vi "FourSessThreePinTwoInstrTwoSiteReservation_CallGetConnectionsFromPinsForOneFgenPinAllSites_ReturnsOneConnection.vi"(8 "error in":errorcluster) -> (0 "error out":errorcluster, 2 "result":string, 3 "pass":bool)   [LabVIEW 2020, in "MeasurementServerTests.lvlib"]
uses:
  MeasurementServerTests.lvlib
  Runtime/MeasurementLink Session Management/Session Reservation/Connection.ctl
  Runtime/MeasurementLink Session Management/Session Reservation/Hardware Independent Connection.ctl
  c3cb69a0-23cd-49fc-99d1-8c54773f0200.vi
  b3e5c3be-b7a7-4b6e-86ee-709eea9cb752.vi
  Runtime/MeasurementLink Session Management/Session Reservation/Get Connections Impl.vi
  Runtime/MeasurementLink Session Management/Session Reservation/Session Reservation.lvclass
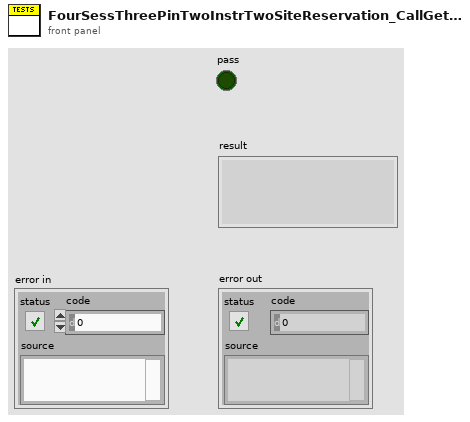
[diagram p1: front panel]
types:
  T1 = typedef "MeasurementLink Session Management.lvlib/Session Reservation.lvclass/Hardware Independent Connection.ctl" = cluster{"pin or relay name":string, "site":i32, "instrument type id":string, "channel":string}
  T2 = typedef "MeasurementLink Session Management.lvlib/Session Reservation.lvclass/Connection.ctl" = cluster{"connection":T1, "session":variant}
  T3 = typedef "MeasurementLink Session Management.lvlib/Session Reservation.lvclass/Data.ctl" = cluster{"session and driver infos":T4[], "pins":string[]}
  T4 = typedef "MeasurementLink Session Management.lvlib/Session Reservation.lvclass/Session and Driver Info.ctl" = cluster{"session info":T5, "session created":bool, "session":variant}
  T5 = typedef "MeasurementLink Session Management Client.lvlib/ni_measurementlink_sessionmanagement_v1_SessionInformation.ctl" = cluster{"session":T6, "resource_name":string, "channel_list":string, "instrument_type_id":string, "session_exists":bool, "channel_mappings":T7[]}
  T6 = typedef "MeasurementLink Session Management Client.lvlib/nidevice_grpc_Session.ctl" = cluster{"name":string}
  T7 = typedef "MeasurementLink Session Management Client.lvlib/ni_measurementlink_sessionmanagement_v1_ChannelMapping.ctl" = cluster{"pin_or_relay_name":string, "site":i32, "channel":string}
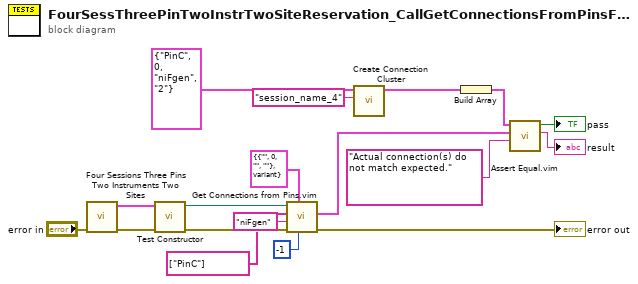
[diagram p0: block diagram]
diagram:
  n1 = call "Four Sessions Three Pins Two Instruments Two Sites.vi"("error in"="error in") -> ("error out"=w7:errorcluster, "data out"=w6:T3)  [unwired: 9 in]
  n2 = call "Test Constructor.vi"("error in"=w7, "data"=w6) -> ("error out"=w17:errorcluster, "Session Reservation out"=w16:refnum<class "Session Reservation.lvclass">)  [unwired: 8 in]
  n3 = call "Get Connections from Pins.vim"("site"=-1, "connection type"=T2 {"connection"={"pin or relay name"="", "site"=0, "instrument type id"="", "channel"=""}, "session"=variant} ("connection"), "error in"=w17, "instrument type id"="niFgen", "pin or relay names"=string[] ["PinC"], "session reservation in"=w16) -> ("error out"=→"error out":errorcluster, "connections"=w13:T2[])  [unwired: 3 in, 1 out]
  n4 = call "Create Connection Cluster.vi"("session in"="session_name_4", "hardware independent connection in"=T1 {"pin or relay name"="PinC", "site"=0, "instrument type id"="niFgen", "channel"="2"} ("connection")) -> ("connection out"=w5:T2)  [unwired: 9 in]
  n5 = Build Array(w5) -> (w4:T2[])
  n6 = call "Assert Equal.vim"("failure message"="Actual connection(s) do not match expected.", "actual value"=w13, "expected value"=w4) -> ("message"=→"result":string, "equal?"=→"pass":bool)  [unwired: 7 in]
